vi "EnqueueMessage.vi"(5 "In Front? (F)":bool, 7 "Timeout (-1 ms)":i32, 8 "error in":errorcluster, 9 "Message Priority (0)":i32, 10 "Message":refnum<class "Message.lvclass">, 11 "PriorityMessageQueue":refnum<class "PriorityMessageQueue.lvclass">) -> (0 "error out":errorcluster, 3 "PriorityMessageQueue out":refnum<class "PriorityMessageQueue.lvclass">, 4 "Timed Out?":bool)   [LabVIEW 2009, in "LapDog.Messaging.v2.lvlib" / "PriorityMessageQueue.lvclass"]
doc: "<b>This class is deprecated in version 2.1 and will be removed in version 3.0</b>\n\nAdds a message to the queue with the given priority. All messages with lower priority numbers are returned from the queue before messages with higher priority numbers."
uses:
  PriorityMessageQueue.lvclass
  MessageObject/Message.lvclass
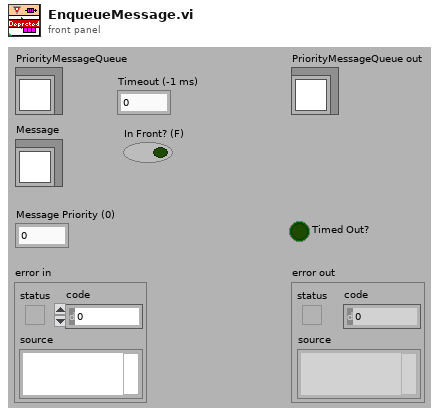
[diagram p1: front panel]
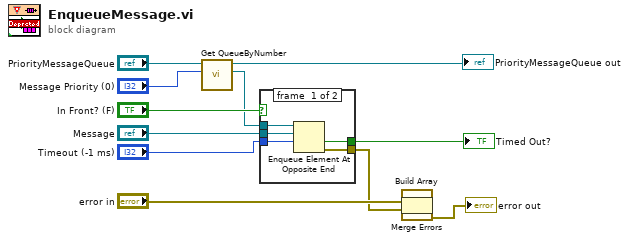
[diagram p0: block diagram]
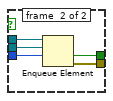
[diagram p2: hidden frame]
diagram:
  n1 = call "Get QueueByNumber.vi"("Priority Level"="Message Priority (0)", "PriorityMessageQueue in"="PriorityMessageQueue") -> ("Message Queue"=w2:refnum<queue>, "PriorityMessageQueue out"=→"PriorityMessageQueue out":refnum<class "PriorityMessageQueue.lvclass">)  [unwired: 8 in]
  n2 = case shown="True" "In Front? (F)" {
    tunnel: w2 -> [w17 w22]
    tunnel: [w16 w21] -> w8
    tunnel: "Message" -> [w15 w20]
    tunnel: "Timeout (-1 ms)" -> [w14 w19]
    tunnel: [w13 w18] -> w6
    frame #0 {
      n3 = Enqueue Element At Opposite End(queue=w17, element=w15, timeout in ms (-1)=w14) -> (timed out?=w13:bool, error out=w16:errorcluster)  [unwired: 1 in, 1 out]
    }
    frame #1 {
      n4 = Enqueue Element(queue=w22, element=w20, timeout in ms (-1)=w19) -> (timed out?=w18:bool, error out=w21:errorcluster)  [unwired: 1 in, 1 out]
    }
  }
  "Timed Out?" <- w6
  n5 = Build Array("error in", w8) -> (w1:errorcluster[])
  n6 = call <vilib>:"Merge Errors.vi"("error array in"=w1) -> ("error out"=→"error out":errorcluster)  [unwired: 6 in]
